vi "Check CCD Config.vi"(8 "error in (no error)":errorcluster, 10 "Status":string, 11 "Channel in":refnum<class "Channel.lvclass">) -> (0 "error out":errorcluster, 1 "cluster RX":T1, 2 "Cluster COMPARE":T2, 3 "Channel out":refnum<class "Channel.lvclass">)   [LabVIEW 2018, in "Channel.lvclass"]
uses:
  Channel.lvclass
  Channel.lvclass/Channel.ctl
panel:
  in  "Cluster CCD conf":cluster{"CCD configuration":string}
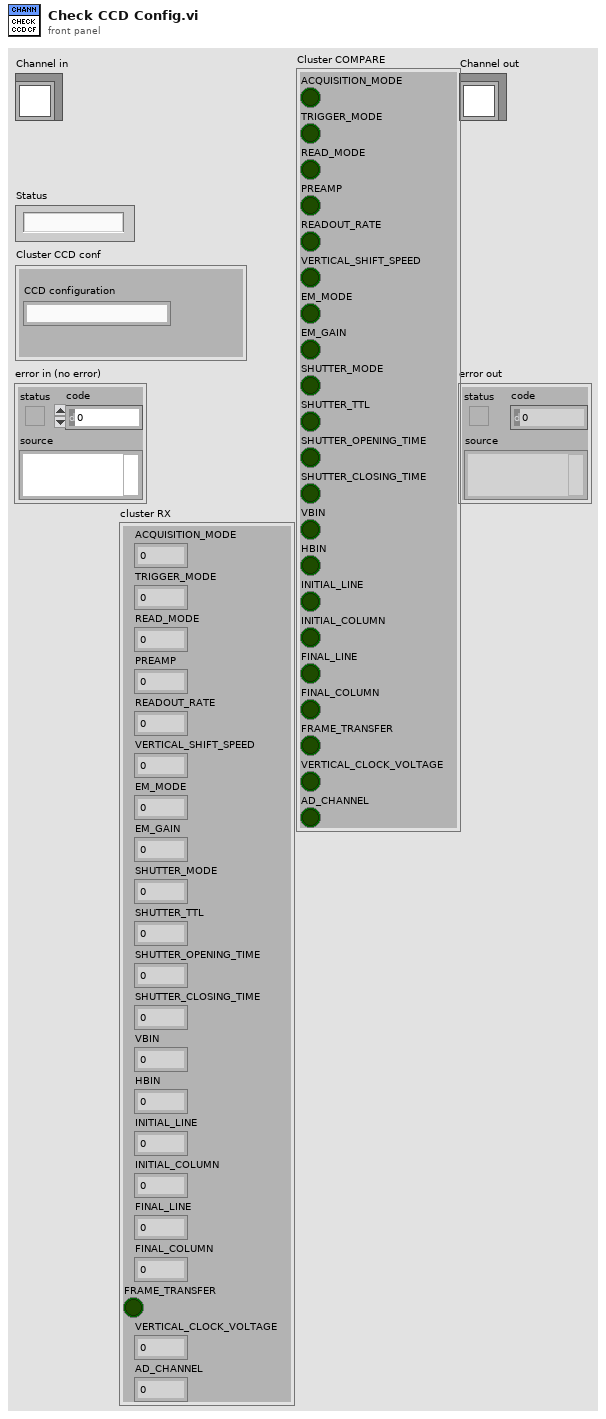
[diagram p1: front panel]
types:
  T1 = cluster{"ACQUISITION_MODE":u8, "TRIGGER_MODE":u8, "READ_MODE":u8, "PREAMP":u8, "READOUT_RATE":u8, "VERTICAL_SHIFT_SPEED":u8, "EM_MODE":u8, "EM_GAIN":u16, "SHUTTER_MODE":u8, "SHUTTER_TTL":u8, "SHUTTER_OPENING_TIME":u16, "SHUTTER_CLOSING_TIME":u16, "VBIN":u16, "HBIN":u16, "INITIAL_LINE":u16, "INITIAL_COLUMN":u16, "FINAL_LINE":u16, "FINAL_COLUMN":u16, "FRAME_TRANSFER":bool, "VERTICAL_CLOCK_VOLTAGE":u8, "AD_CHANNEL":u32}
  T2 = cluster{"ACQUISITION_MODE":bool, "TRIGGER_MODE":bool, "READ_MODE":bool, "PREAMP":bool, "READOUT_RATE":bool, "VERTICAL_SHIFT_SPEED":bool, "EM_MODE":bool, "EM_GAIN":bool, "SHUTTER_MODE":bool, "SHUTTER_TTL":bool, "SHUTTER_OPENING_TIME":bool, "SHUTTER_CLOSING_TIME":bool, "VBIN":bool, "HBIN":bool, "INITIAL_LINE":bool, "INITIAL_COLUMN":bool, "FINAL_LINE":bool, "FINAL_COLUMN":bool, "FRAME_TRANSFER":bool, "VERTICAL_CLOCK_VOLTAGE":bool, "AD_CHANNEL":bool}
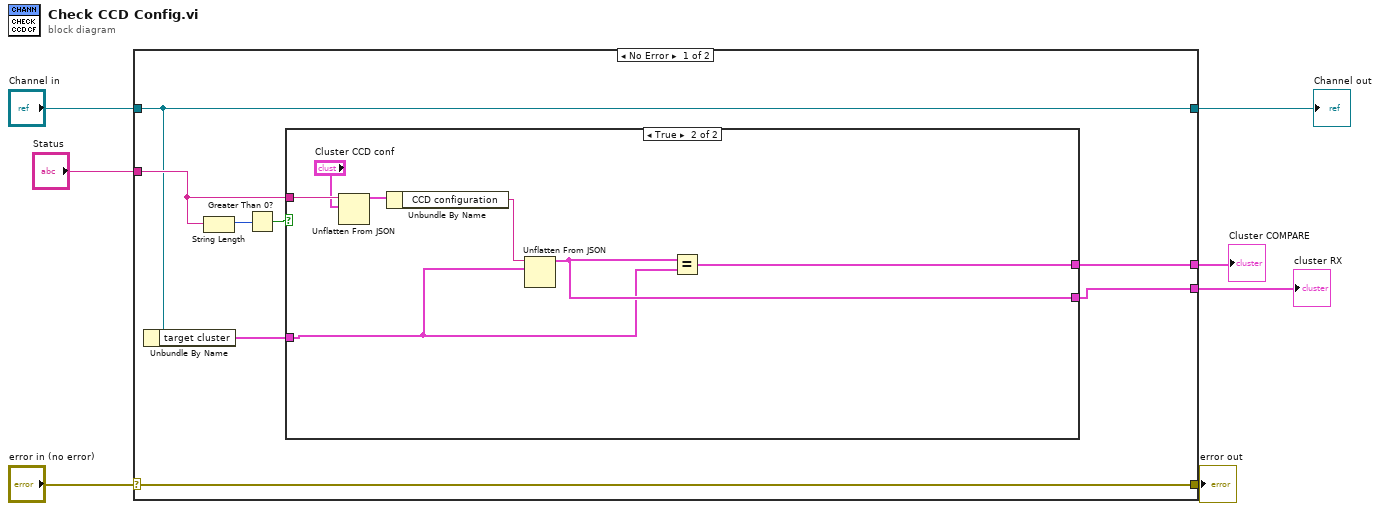
[diagram p0: block diagram]
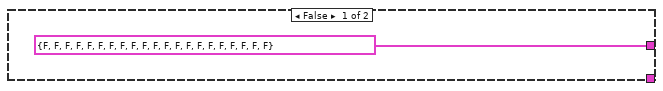
[diagram p2: hidden frame]
diagram:
  n1 = case shown="No Error" "error in (no error)" {
    selector: "error in (no error)" -> [w15 w25]
    tunnel: [w15 w25] -> w6
    tunnel: [w11 w24] -> w4
    tunnel: "Channel in" -> [w11 w24]
    tunnel: "Status" -> [w13 _]
    tunnel: [w9 _] -> w2
    tunnel: [w8 _] -> w1
    frame No Error {
      n2 = Unbundle By Name(w11) -> ("target cluster"=w10:T1)
      n3 = String Length(string=w13) -> (length=w14:i32)
      n4 = Greater Than 0?(x=w14) -> (x > 0?=w12:bool)
      n5 = case shown="True" w12 {
        tunnel: w13 -> [_ w23]
        tunnel: [T2 {"ACQUISITION_MODE"=FALSE, "TRIGGER_MODE"=FALSE, "READ_MODE"=FALSE, "PREAMP"=FALSE, "READOUT_RATE"=FALSE, "VERTICAL_SHIFT_SPEED"=FALSE, "EM_MODE"=FALSE, "EM_GAIN"=FALSE, "SHUTTER_MODE"=FALSE, "SHUTTER_TTL"=FALSE, "SHUTTER_OPENING_TIME"=FALSE, "SHUTTER_CLOSING_TIME"=FALSE, "VBIN"=FALSE, "HBIN"=FALSE, "INITIAL_LINE"=FALSE, "INITIAL_COLUMN"=FALSE, "FINAL_LINE"=FALSE, "FINAL_COLUMN"=FALSE, "FRAME_TRANSFER"=FALSE, "VERTICAL_CLOCK_VOLTAGE"=FALSE, "AD_CHANNEL"=FALSE} w19] -> w9
        tunnel: [_ w18] -> w8
        tunnel: w10 -> [_ w17]
        frame False {
        }
        frame True {
          n6 = Unflatten From JSON(JSON string=w23, type and defaults="Cluster CCD conf") -> (value=w21:cluster{"CCD configuration":string})  [unwired: 5 in, 1 out]
          n7 = Unbundle By Name(w21) -> ("CCD configuration"=w20:string)
          n8 = Unflatten From JSON(JSON string=w20, type and defaults=w17) -> (value=w18:T1)  [unwired: 5 in, 1 out]
          n9 = Equal?(x=w18, y=w17) -> (x = y?=w19:T2)
        }
      }
    }
    frame Error {
    }
  }
  "error out" <- w6
  "Channel out" <- w4
  "Cluster COMPARE" <- w2
  "cluster RX" <- w1
